vi "ESC Set RPM With Feedback.vi"(6 "Calib File":path, 8 "Meas Setup filename":string, 11 "Desired RPM":dbl min=0.0 max=32500.0) -> (0 "Error Out":errorcluster, 2 "Meas RPM":dbl, 3 "PWM%":dbl)   [LabVIEW 2022 SP3]
uses:
  Anemometry/Anemometry Sub Vis/File/Setup_Filetype.ctl
  Anemometry/Anemometry Sub Vis/Controls/Setup.ctl
  Anemometry/Anemometry Sub Vis/Controls/Save_Data.ctl
  Anemometry/Anemometry Sub Vis/Gen Trav/Multi_Run_Status.ctl
  Anemometry/Anemometry Sub Vis/Globals/Meas_global.vi
  Anemometry/Anemometry Sub Vis/Globals/Dynamic_call_global.ph.vi
  <vilib>/Analysis/NI_AALPro.lvlib
panel:
  in  "stop":bool
  out "Iteration No":i32
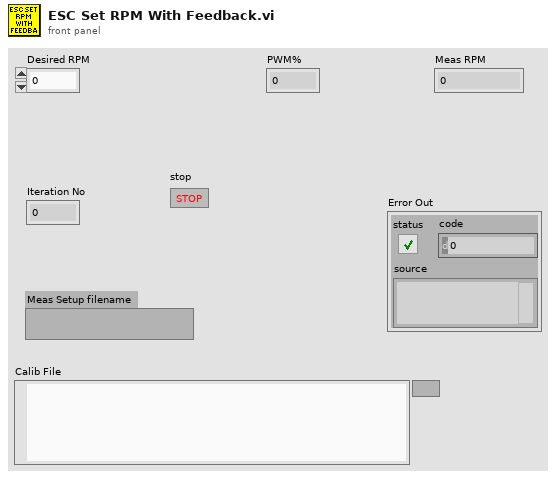
[diagram p1: front panel]
types:
  T1 = typedef "Setup_Filetype.ctl" = enum16{"Measurement Setups", "Calibration Setups", "General", "Results File Plotter Setups", "Speed Calib Tweaks"}
  T2 = enum16{"Zero or one", "One", "Zero or more", "One or more"}
  T3 = typedef "Save_Data.ctl" = enum16{"Save No Data", "Save Data"}
  T4 = typedef "Setup.ctl" = enum16{"Run Program", "Show Setup", "Save Current Setup", "Setup Front Panel"}
  T5 = typedef "Multi_Run_Status.ctl" = enum16{"Continue", "Continue with Error", "Jump to Next Point", "Jump to Next Row", "Jump To Fall Back", "Terminate Run"}
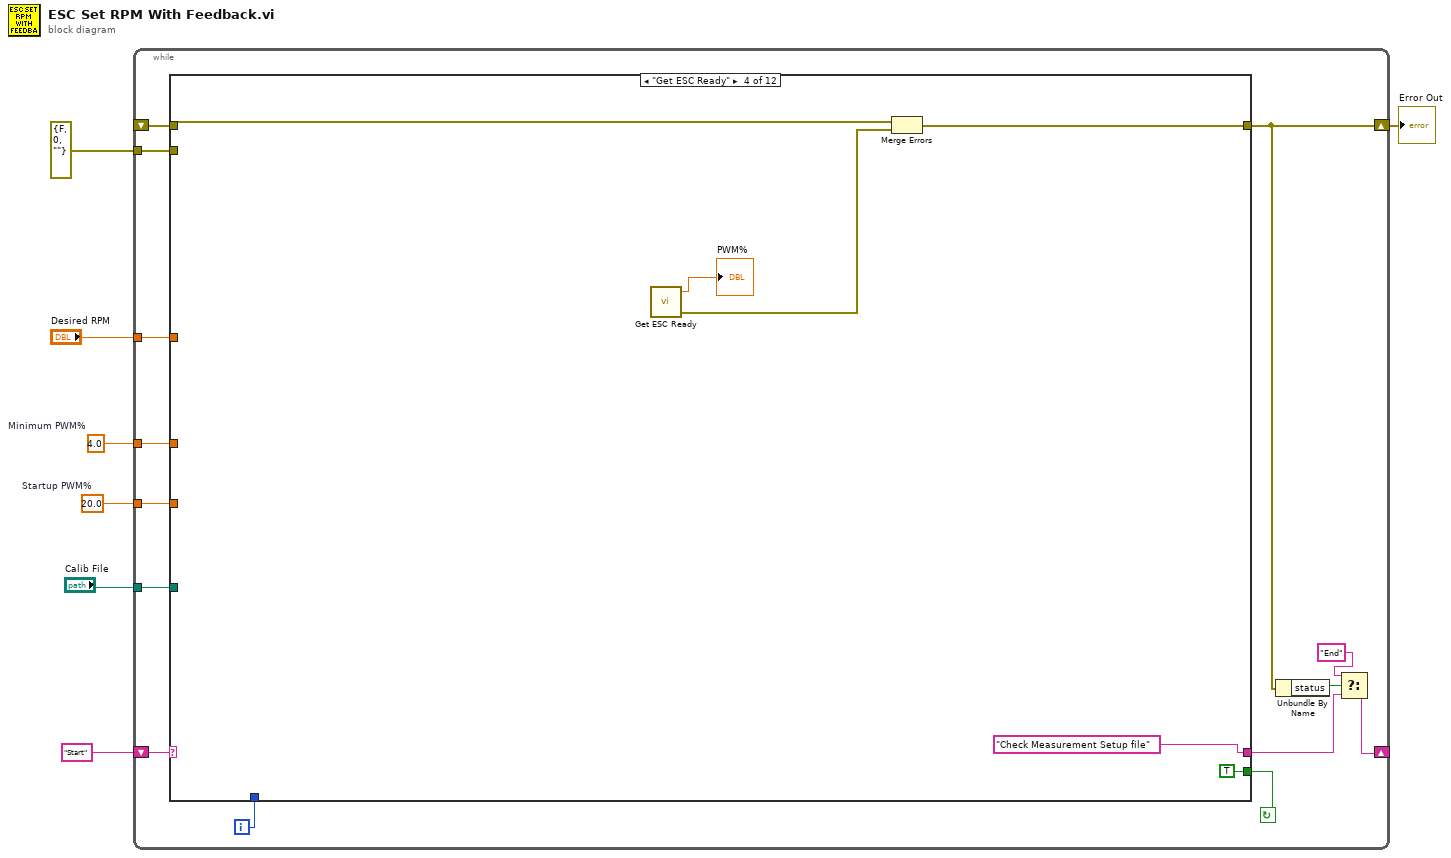
[diagram p0: block diagram]
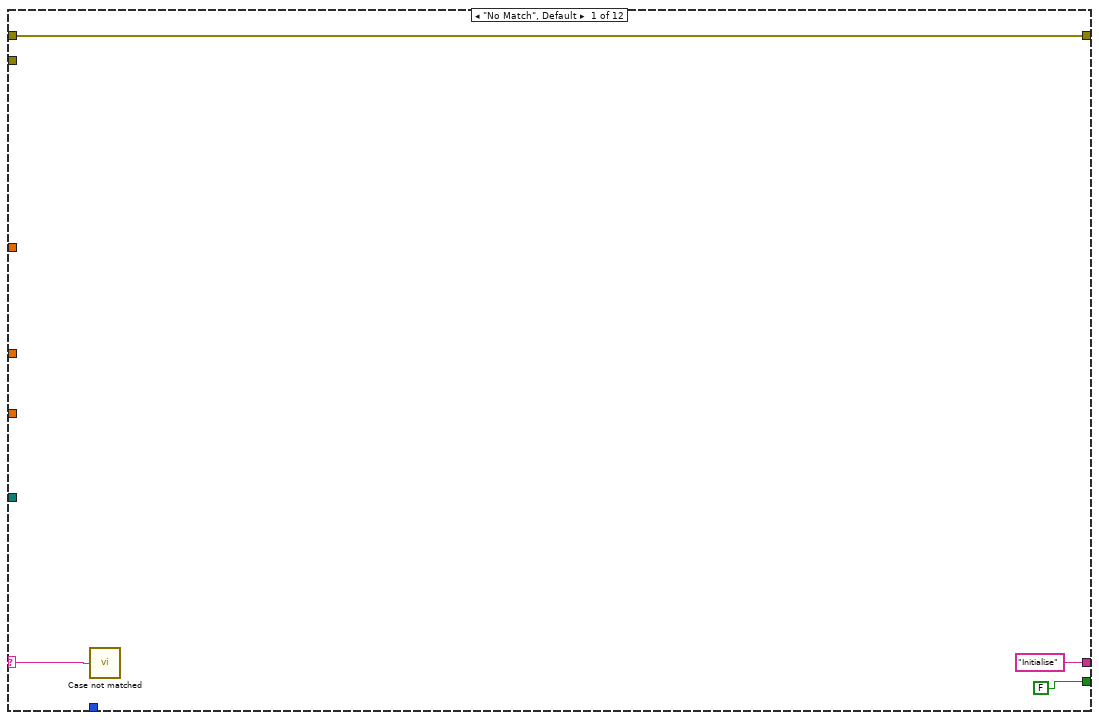
[diagram p2: hidden frame]
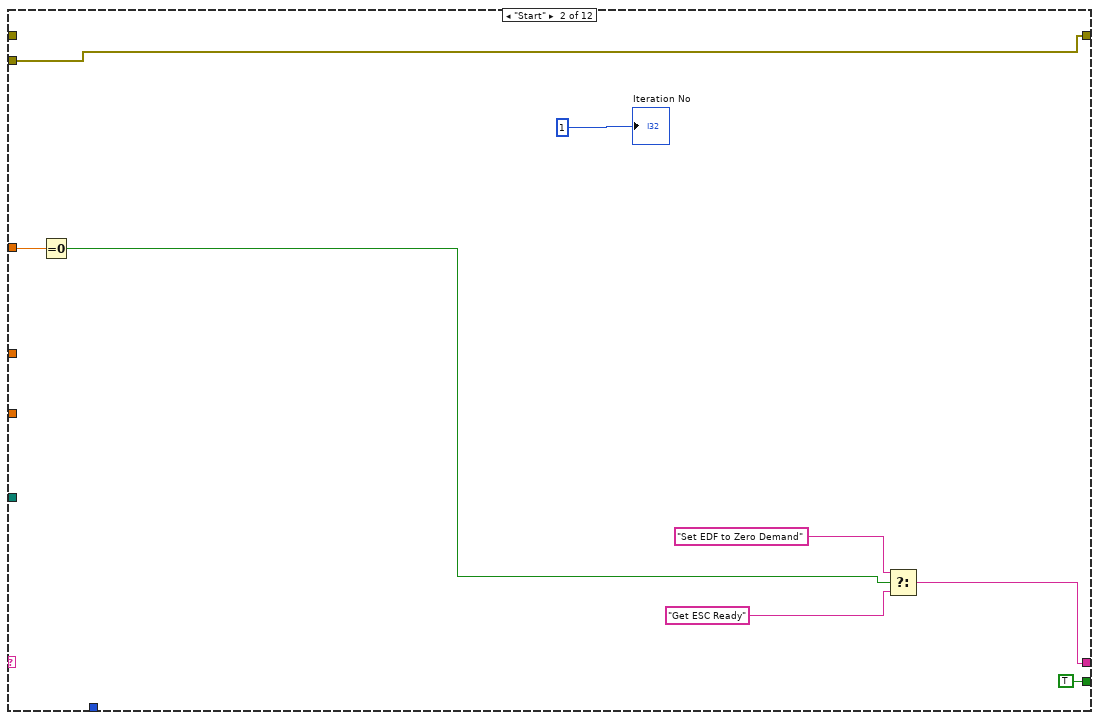
[diagram p3: hidden frame]
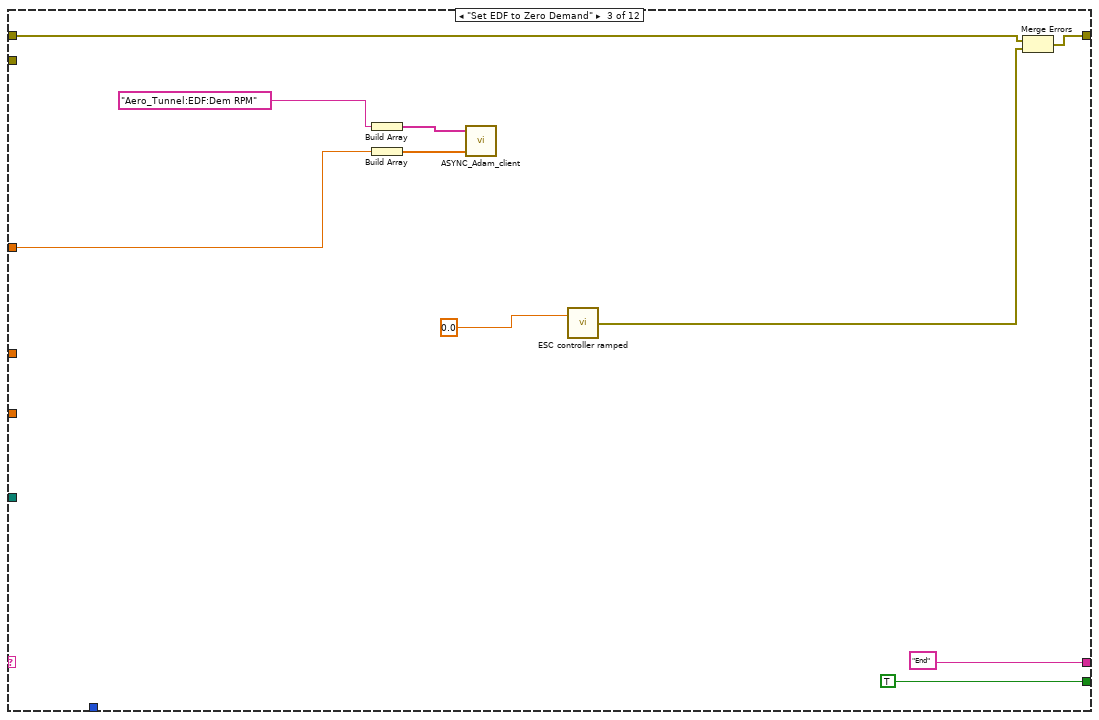
[diagram p4: hidden frame]
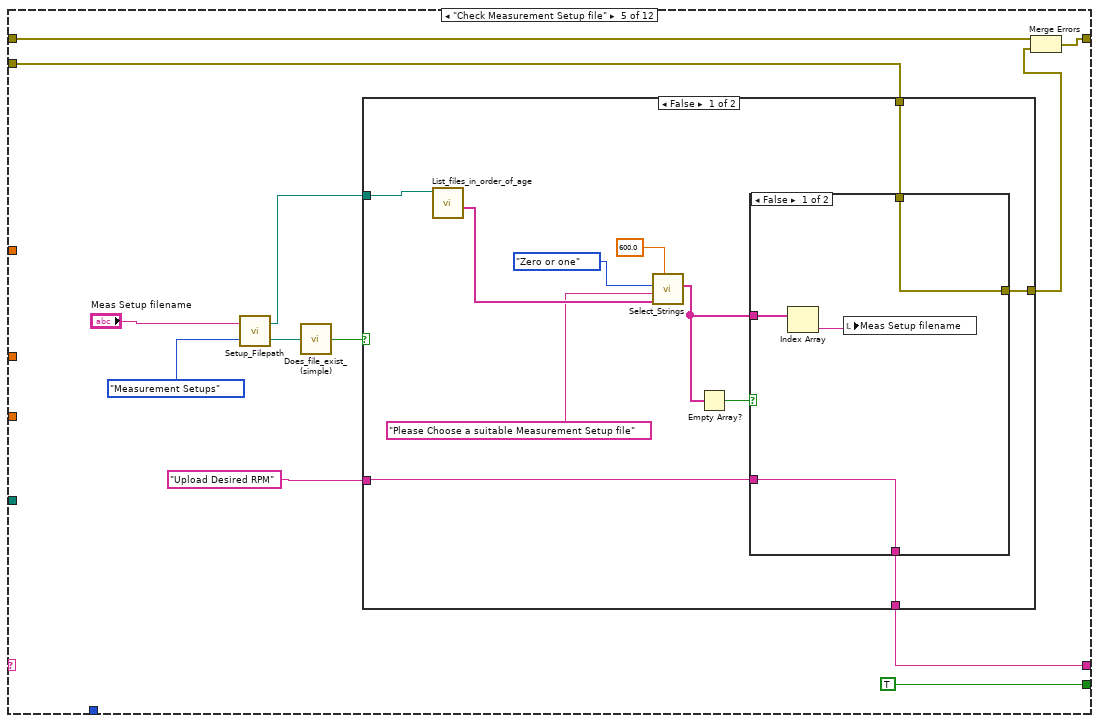
[diagram p5: hidden frame]
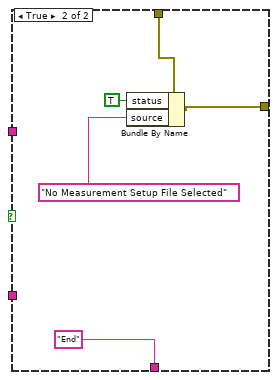
[diagram p6: hidden frame]
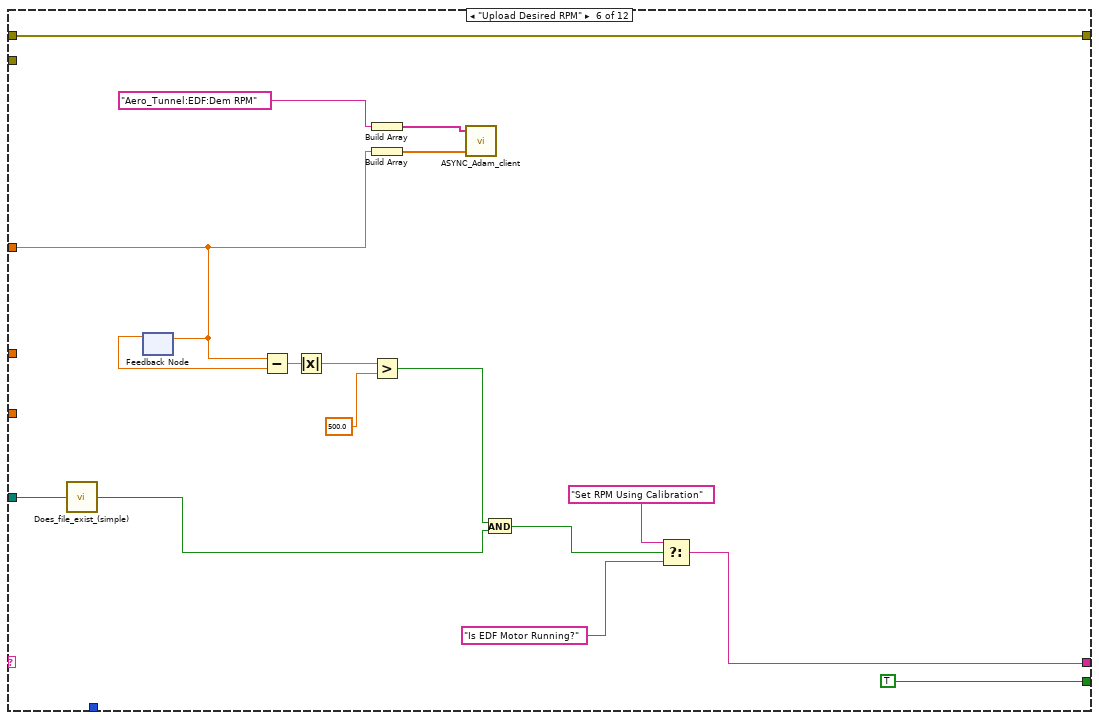
[diagram p8: hidden frame]
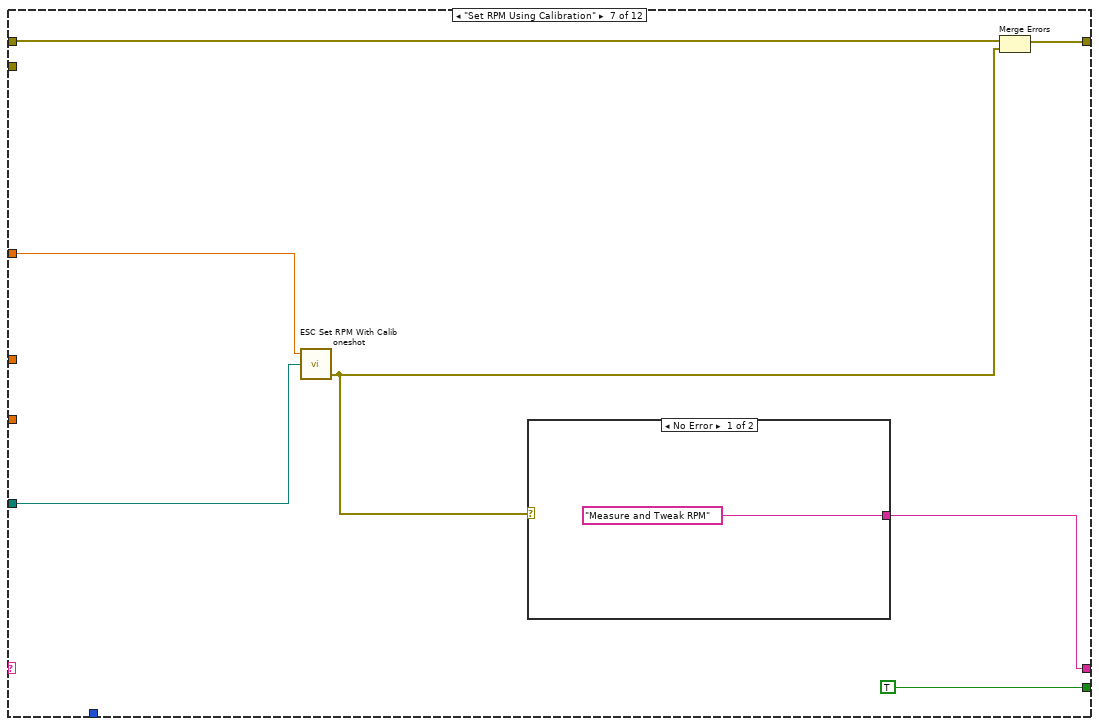
[diagram p9: hidden frame]
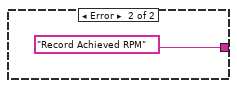
[diagram p10: hidden frame]
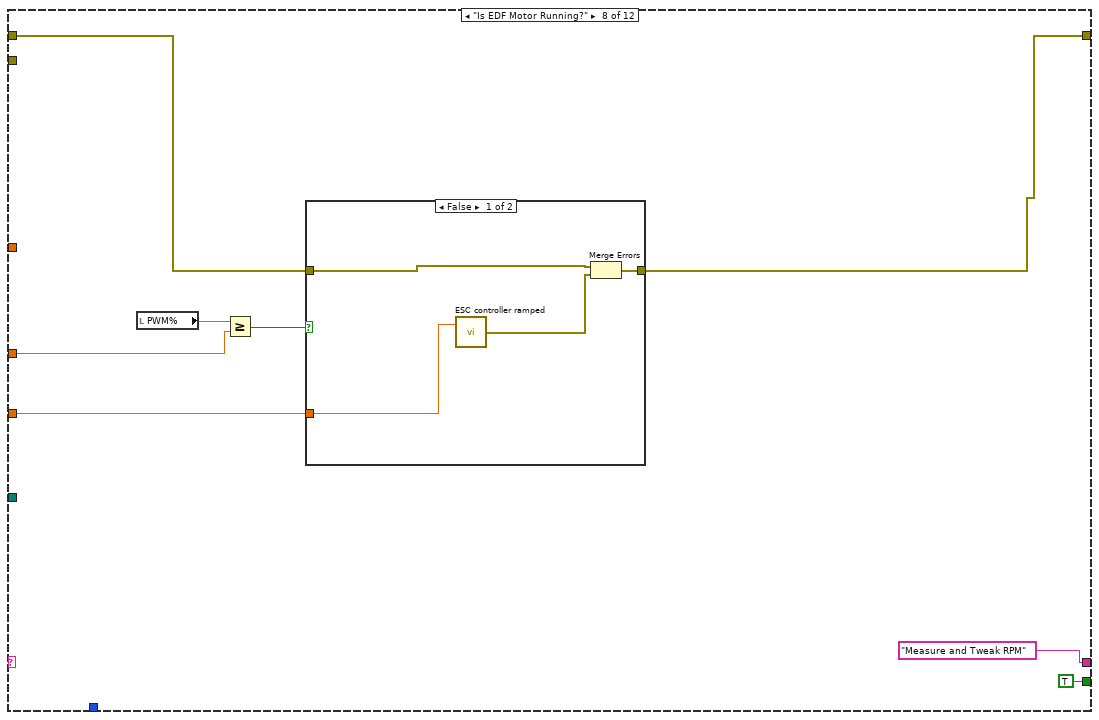
[diagram p11: hidden frame]
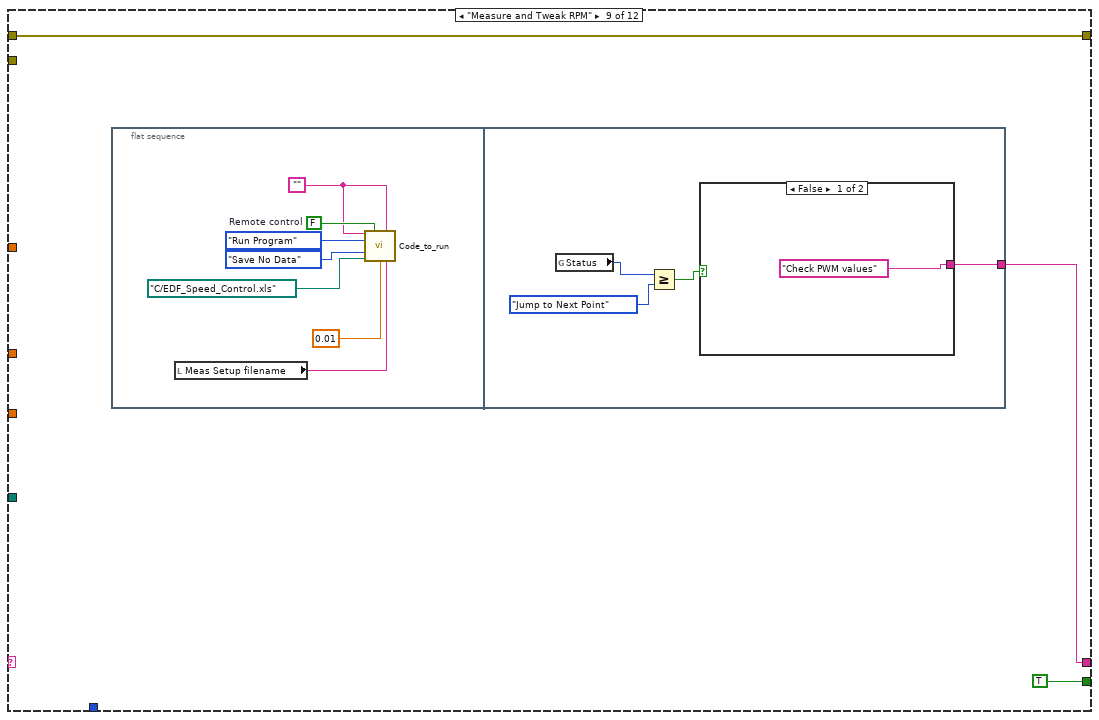
[diagram p13: hidden frame]
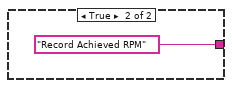
[diagram p14: hidden frame]
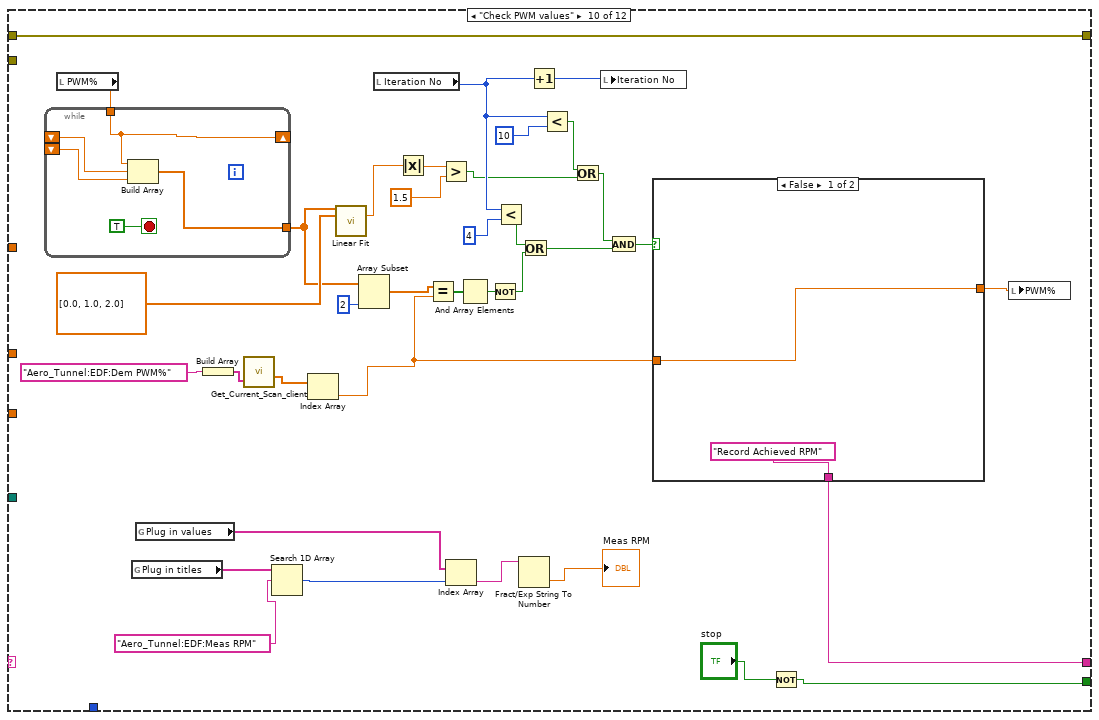
[diagram p15: hidden frame]
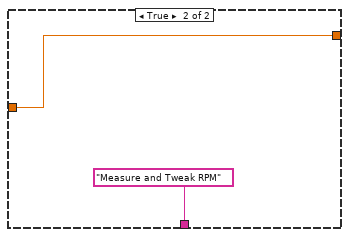
[diagram p16: hidden frame]
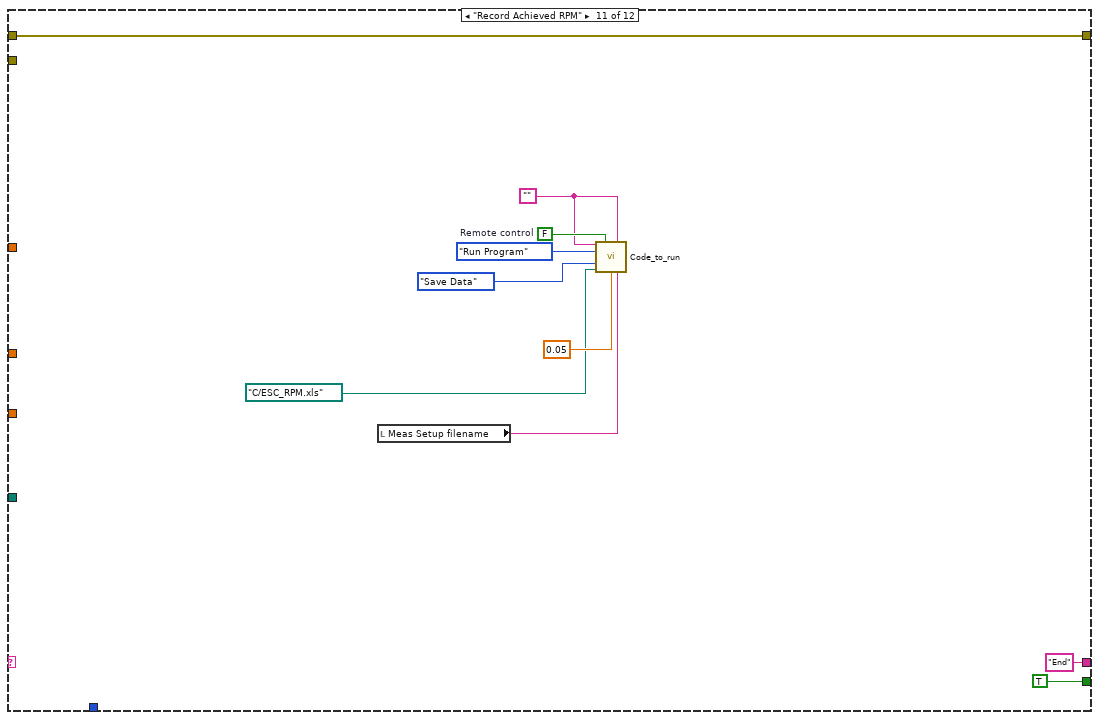
[diagram p17: hidden frame]
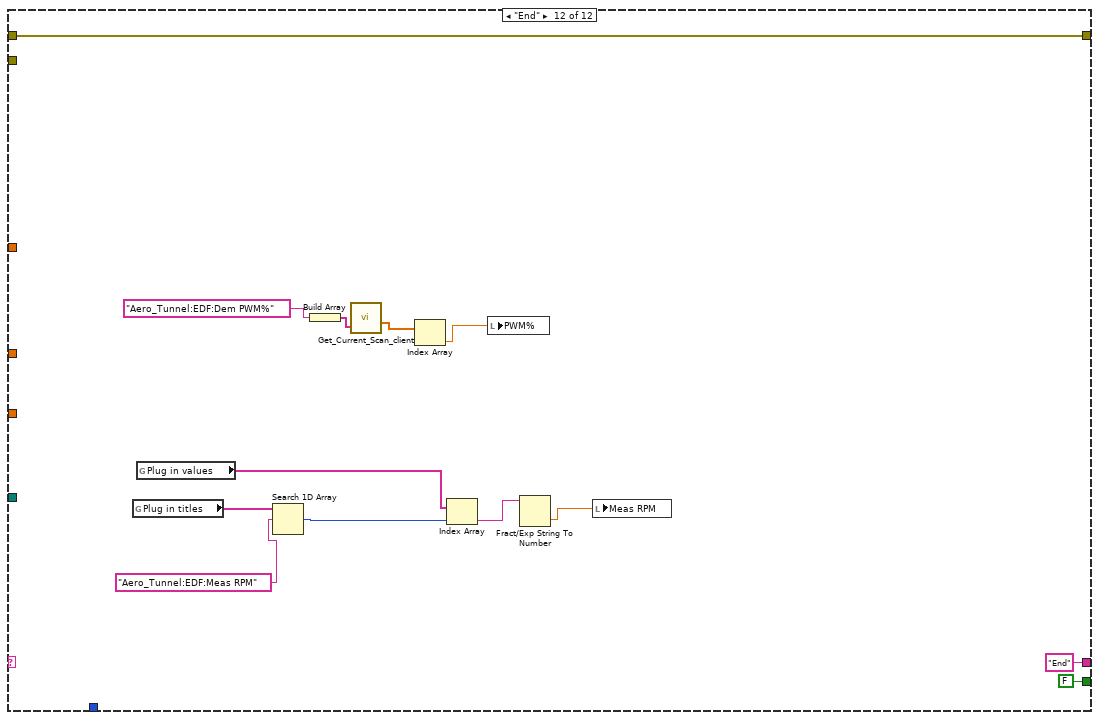
[diagram p18: hidden frame]
diagram:
  w1 = 20.0  # Startup PWM%
  w2 = 4.0  # Minimum PWM%
  n1 = while {
    shift-left: "Start" -> [w20]
    shift-right: [w10] -> _
    shift-right: [w12] -> w3
    shift-left: _ -> [w19]
    tunnel: "Desired RPM" -> [w17]
    tunnel: "Calib File" -> [w16]
    tunnel: errorcluster {"status"=FALSE, "code"=0, "source"=""} ("error IO") -> [w15]
    tunnel: w2 -> [w9]
    tunnel: w1 -> [w8]
    i -> [w18]
    stop <- w21 continue-if-true
    n2 = case shown="\"Get ESC Ready\"" w20 {
      selector: w20 -> [w23 _ _ _ _ _ _ _ _ _ _ _]
      tunnel: [FALSE TRUE TRUE TRUE TRUE TRUE TRUE TRUE TRUE w139 TRUE FALSE] -> w21
      tunnel: ["Initialise" w29 "End" "Check Measurement Setup file" w55 w93 w104 "Measure and Tweak RPM" w123 w173 "End" "End"] -> w11
      tunnel: [w22 w26 w35 w47 w50 w96 w102 w113 w124 w172 w187 w206] -> w12
      tunnel: w19 -> [w22 _ w34 w49 w52 w96 w103 w115 w124 w172 w187 w206]
      tunnel: w18 -> [_ _ _ _ _ _ _ _ _ _ _ _]
      tunnel: w17 -> [_ w33 w38 _ _ w91 w105 _ _ _ _ _]
      tunnel: w16 -> [_ _ _ _ _ w95 w106 _ _ _ _ _]
      tunnel: w15 -> [_ w26 _ _ w53 _ _ _ _ _ _ _]
      tunnel: w9 -> [_ _ _ _ _ _ _ w111 _ _ _ _]
      tunnel: w8 -> [_ _ _ _ _ _ _ w110 _ _ _ _]
      frame "No Match", Default {
        n3 = call "Case not matched.vi"("Case Name not Matched"=w23) -> ()
      }
      frame "Start" {
        n4 = Equal To 0?(x=w33) -> (x = 0?=w31:bool)
        n5 = Select(t="Set EDF to Zero Demand", s=w31, f="Get ESC Ready") -> (s? t:f=w29:string)
        "Iteration No" <- 1 ("Iteration No")
      }
      frame "Set EDF to Zero Demand" {
        n6 = Build Array("Aero_Tunnel:EDF:Dem RPM") -> (w39:string[])
        n7 = Build Array(w38) -> (w41:dbl[])
        n8 = call "ASYNC_Adam_client.vi"("Values"=w41, "Channel Names"=w39) -> ()  [unwired: 1 in, 2 out]
        n9 = call "ESC controller ramped.vi"("Output %"=sgl 0.0) -> ("Error out"=w36:errorcluster)  [unwired: 2 in]
        n10 = Merge Errors(w34, w36) -> (w35:errorcluster)
      }
      frame "Get ESC Ready" {
        n11 = call "Get ESC Ready.vi"() -> ("Error out"=w48:errorcluster, "Current PWM%"=→"PWM%":dbl)  [unwired: 4 in]
        n12 = Merge Errors(w49, w48) -> (w47:errorcluster)
      }
      frame "Check Measurement Setup file" {
        n13 = call "Setup_Filepath.vi"("Setup File Type"=Setup_Filetype."Measurement Setups", "Filename in"="Meas Setup filename") -> ("Filename Out"=w60:path, "Directory"=w58:path)
        n14 = call "Does_file_exist_(simple).vi"("Pathname"=w60) -> ("exists?"=w57:bool)
        n15 = case shown="False" w57 {
          tunnel: w58 -> [w72 _]
          tunnel: [w67 w83] -> w55
          tunnel: "Upload Desired RPM" -> [w66 w83]
          tunnel: w53 -> [w63 w82]
          tunnel: [w62 w82] -> w51
          frame False {
            n16 = call "List_files_in_order_of_age.vi"("Folder"=w72) -> ("file names"=w70:string[])  [unwired: 10 in]
            n17 = call "Select_Strings.vi"("Timeout (s)"=600.0, "Available Ch names"=w70, "Message"="Please Choose a suitable Measurement Setup file", "Selector mode"=T2."Zero or one") -> ("Selected Channel Names"=w65:string[])  [unwired: 2 in, 2 out]
            n18 = Empty Array?(array=w65) -> (empty?=w68:bool)
            n19 = case shown="False" w68 {
              tunnel: [w76 "End"] -> w67
              tunnel: w66 -> [w76 _]
              tunnel: w65 -> [w75 _]
              tunnel: w63 -> [w73 w80]
              tunnel: [w73 w77] -> w62
              frame False {
                n20 = Index Array(array=w75) -> (element=w74:string)  [unwired: 1 in]
                n21 = local write "Meas Setup filename"(w74) -> ()
              }
              frame True {
                n22 = Bundle By Name(cluster=w80, "status"=TRUE, "source"="No Measurement Setup File Selected") -> (w77:errorcluster)
              }
            }
          }
          frame True {
          }
        }
        n23 = Merge Errors(w52, w51) -> (w50:errorcluster)
      }
      frame "Upload Desired RPM" {
        n24 = call "Does_file_exist_(simple).vi"("Pathname"=w95) -> ("exists?"=w85:bool)
        n25 = feedback-in #1(w91) -> ()
        n26 = feedback #1() -> (w90:dbl)  [unwired: 1 in]
        n27 = Subtract(x=w91, y=w90) -> (x-y=w89:dbl)
        n28 = Absolute Value(x=w89) -> (abs(x)=w88:dbl)
        n29 = Build Array("Aero_Tunnel:EDF:Dem RPM") -> (w97:string[])
        n30 = Build Array(w91) -> (w99:dbl[])
        n31 = Greater?(x=w88, y=500.0) -> (0:w86:bool)
        n32 = call "ASYNC_Adam_client.vi"("Values"=w99, "Channel Names"=w97) -> ()  [unwired: 1 in, 2 out]
        n33 = And(x=w86, y=w85) -> (x .and. y?=w84:bool)
        n34 = Select(t="Set RPM Using Calibration", s=w84, f="Is EDF Motor Running?") -> (s? t:f=w93:string)
      }
      frame "Set RPM Using Calibration" {
        n35 = call "ESC Set RPM With Calib oneshot.vi"("Calib File"=w106, "Desired RPM"=w105) -> ("Error out"=w101:errorcluster)  [unwired: 2 in, 1 out]
        n36 = case shown="No Error" w101 {
          tunnel: ["Measure and Tweak RPM" "Record Achieved RPM"] -> w104
          frame No Error {
          }
          frame Error {
          }
        }
        n37 = Merge Errors(w103, w101) -> (w102:errorcluster)
      }
      frame "Is EDF Motor Running?" {
        n38 = local read "PWM%"() -> (w117:dbl)
        n39 = Greater Or Equal?(x=w117, y=w111) -> (x >= y?=w116:bool)
        n40 = case shown="False" w116 {
          tunnel: [w119 w122] -> w113
          tunnel: w115 -> [w121 w122]
          tunnel: w110 -> [w118 _]
          frame False {
            n41 = call "ESC controller ramped.vi"("Output %"=w118) -> ("Error out"=w120:errorcluster)  [unwired: 2 in]
            n42 = Merge Errors(w121, w120) -> (w119:errorcluster)
          }
          frame True {
          }
        }
      }
      frame "Measure and Tweak RPM" {
        n43 = flat-sequence {
          tunnel: [w133] -> w123
          frame #0 {
            w129 = ""
            w130 = FALSE  # Remote control
            n44 = local read "Meas Setup filename"() -> (w126:string)
            n45 = call "Code_to_run.vi"("Extra command String"=w129, "Current Row Comments"=w129, "setup"=Setup."Run Program", "Remote control"=w130, "File"=Save_Data."Save No Data", "Results Filename"=path "C:/EDF_Speed_Control.xls", "Averaging time (min)"=0.01, "Setup filename"=w126) -> ()  [unwired: 4 in, 4 out]
          }
          frame #1 {
            n46 = global read "Meas_global.vi" "Status"() -> (w136:T5)
            n47 = Greater Or Equal?(x=w136, y=Multi_Run_Status."Jump to Next Point" ("Status")) -> (x >= y?=w134:bool)
            n48 = case shown="False" w134 {
              tunnel: ["Check PWM values" "Record Achieved RPM"] -> w133
              frame False {
              }
              frame True {
              }
            }
          }
        }
      }
      frame "Check PWM values" {
        n49 = local read "PWM%"() -> (w170:dbl)
        n50 = while {
          shift-right: [w177] -> _
          shift-left: _ -> [w179]
          tunnel: w170 -> [w177]
          tunnel: [w176] -> w149
          shift-left: _ -> [w175]
          stop <- TRUE stop-if-true
          n51 = Build Array(w177, w179, w175) -> (w176:dbl[])
        }
        n52 = global read "Dynamic_call_global.ph.vi" "Plug in titles"() -> (w146:string[])
        n53 = global read "Dynamic_call_global.ph.vi" "Plug in values"() -> (w144:string[])
        n54 = Build Array("Aero_Tunnel:EDF:Dem PWM%") -> (w161:string[])
        n55 = call "Get_Current_Scan_client.vi"("multipleChannels"=w161) -> ("Numerical Values"=w174:dbl[])  [unwired: 1 in, 3 out]
        n56 = Search 1D Array(1D array=w146, element="Aero_Tunnel:EDF:Meas RPM" ("string")) -> (index of element=w143:i32)  [unwired: 1 in]
        n57 = Index Array(array=w174) -> (element=w168:dbl)  [unwired: 1 in]
        n58 = call <vilib>:"Linear Fit.vi"("Y"=w149, "X"=dbl[] [0.0, 1.0, 2.0]) -> ("slope"=w150:dbl)  [unwired: 9 in, 4 out]
        n59 = Array Subset(array=w149, length=2) -> (w148:dbl[])  [unwired: 1 in]
        n60 = local read "Iteration No"() -> (w160:i32)
        n61 = Absolute Value(x=w150) -> (abs(x)=w156:dbl)
        n62 = Equal?(x=w148, y=w168) -> (x = y?=w169:bool[])
        n63 = Greater?(x=w156, y=1.5) -> (0:w153:bool)
        n64 = Index Array(array=w144, index=w143) -> (element=w142:string)
        n65 = And Array Elements(Boolean array=w169) -> (logical AND=w165:bool)
        n66 = Not(x=w165) -> (.not. x?=w163:bool)
        n67 = Less?(x=w160, y=4) -> (x < y?=w164:bool)
        n68 = Fract/Exp String To Number(string=w142) -> (number=→"Meas RPM":dbl)  [unwired: 3 in, 1 out]
        n69 = Or(x=w164, y=w163) -> (x .or. y?=w158:bool)
        n70 = Increment(x=w160) -> (x+1=w167:i32)
        n71 = Less?(x=w160, y=10) -> (x < y?=w154:bool)
        n72 = Or(x=w154, y=w153) -> (x .or. y?=w152:bool)
        n73 = local write "Iteration No"(w167) -> ()
        n74 = And(x=w152, y=w158) -> (x .and. y?=w157:bool)
        n75 = case shown="False" w157 {
          tunnel: ["Record Achieved RPM" "Measure and Tweak RPM"] -> w173
          tunnel: [w180 w182] -> w171
          tunnel: w168 -> [w180 w182]
          frame False {
          }
          frame True {
          }
        }
        n76 = Not(x="stop") -> (.not. x?=w139:bool)
        n77 = local write "PWM%"(w171) -> ()
      }
      frame "Record Achieved RPM" {
        w189 = ""
        w190 = FALSE  # Remote control
        n78 = local read "Meas Setup filename"() -> (w184:string)
        n79 = call "Code_to_run.vi"("Extra command String"=w189, "Current Row Comments"=w189, "setup"=Setup."Run Program", "Remote control"=w190, "File"=Save_Data."Save Data", "Results Filename"=path "C:/ESC_RPM.xls", "Averaging time (min)"=0.05, "Setup filename"=w184) -> ()  [unwired: 4 in, 4 out]
      }
      frame "End" {
        n80 = global read "Dynamic_call_global.ph.vi" "Plug in titles"() -> (w199:string[])
        n81 = global read "Dynamic_call_global.ph.vi" "Plug in values"() -> (w197:string[])
        n82 = Search 1D Array(1D array=w199, element="Aero_Tunnel:EDF:Meas RPM" ("string")) -> (index of element=w196:i32)  [unwired: 1 in]
        n83 = Build Array("Aero_Tunnel:EDF:Dem PWM%") -> (w201:string[])
        n84 = call "Get_Current_Scan_client.vi"("multipleChannels"=w201) -> ("Numerical Values"=w203:dbl[])  [unwired: 1 in, 3 out]
        n85 = Index Array(array=w203) -> (element=w200:dbl)  [unwired: 1 in]
        n86 = Index Array(array=w197, index=w196) -> (element=w195:string)
        n87 = local write "PWM%"(w200) -> ()
        n88 = Fract/Exp String To Number(string=w195) -> (number=w194:dbl)  [unwired: 3 in, 1 out]
        n89 = local write "Meas RPM"(w194) -> ()
      }
    }
    n90 = Unbundle By Name(w12) -> ("status"=w14:bool)
    n91 = Select(t="End", s=w14, f=w11) -> (s? t:f=w10:string)
  }
  "Error Out" <- w3
